vi "Write File (Complete).vi"(8 "error in (no error)":errorcluster, 10 "String":string, 11 "ConfigManager.Text in":refnum<class "ConfigManager.Text.lvclass">) -> (0 "error out":errorcluster, 3 "ConfigManager.Text out":refnum<class "ConfigManager.Text.lvclass">)   [LabVIEW 2013, in "CfgManager.Text.lvlib" / "ConfigManager.Text.lvclass"]
uses:
  ConfigManager.Text.lvclass
  ConfigManager.Text.lvclass/ConfigManager.Text.ctl
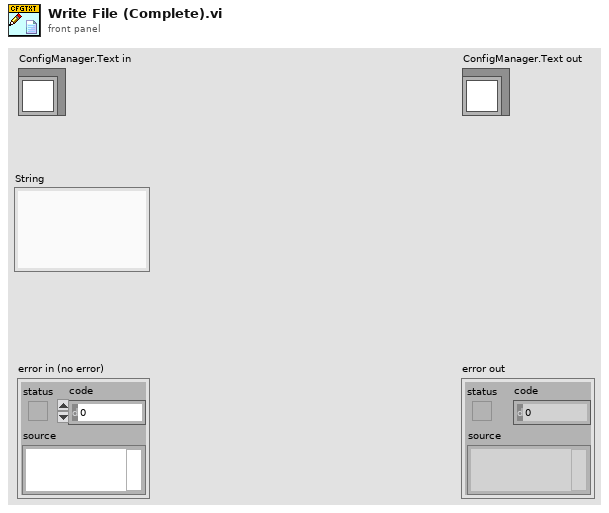
[diagram p1: front panel]
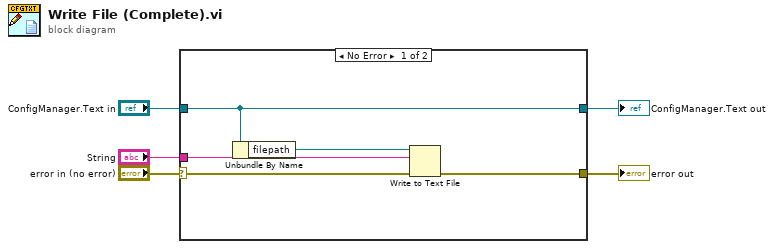
[diagram p0: block diagram]
diagram:
  n1 = case shown="No Error" "error in (no error)" {
    selector: "error in (no error)" -> [w8 w12]
    tunnel: [w7 w12] -> w4
    tunnel: [w9 w11] -> w2
    tunnel: "ConfigManager.Text in" -> [w9 w11]
    tunnel: "String" -> [w6 _]
    frame No Error {
      n2 = Unbundle By Name(w9) -> ("filepath"=w10:path)
      n3 = Write to Text File(file (use dialog)=w10, text=w6, error in=w8) -> (error out=w7:errorcluster)  [unwired: 1 in, 2 out]
    }
    frame Error {
    }
  }
  "error out" <- w4
  "ConfigManager.Text out" <- w2
